vi "My Schedule vs Prins FIFO Scheduler with Plotting.vi"() -> ()   [LabVIEW 2013, in "Scheduler.lvclass"]
uses:
  Scheduler.lvclass
  Controls/GanntChart_Element.ctl
  Controls/GapStructure4FIFOEngine.ctl
  Controls/Prins FIFO Scheduler Result Cluster.ctl
  Operation to Machine Job Tuple.vi
  Check Other Machines for Schedule Time.vi
  Schedule Job.vi
  Find Gaps on Particular Machine.vi
  Increment Number of Jobs on Machine.vi
  Find Job On Other Machines.vi
  <vilib>/dlg_ctls.llb/Space Constant.vi
  <vilib>/Analysis/1siggen.llb/Riffle Array (I32).vi
  <vilib>/Heliosphere Research LLC/Advanced Plotting Toolkit/api_core/New.vi
  <vilib>/Heliosphere Research LLC/Advanced Plotting Toolkit/api_annotations/XLabel.vi
  <vilib>/Heliosphere Research LLC/Advanced Plotting Toolkit/api_figure/YTicks.vi
  <vilib>/Heliosphere Research LLC/Advanced Plotting Toolkit/api_figure/Grids.vi
  <vilib>/Heliosphere Research LLC/Advanced Plotting Toolkit/api_core/View.vi
  <vilib>/Heliosphere Research LLC/Advanced Plotting Toolkit/api_core/Close.vi
  <vilib>/Heliosphere Research LLC/Advanced Plotting Toolkit/api_figure/Limits.vi
  <vilib>/Heliosphere Research LLC/Advanced Plotting Toolkit/api_annotations/Rectangle.vi
  <vilib>/Heliosphere Research LLC/Advanced Plotting Toolkit/api_annotations/Text.vi
  <vilib>/Analysis/NI_AALBase.lvlib
panel:
  out "Total Tardiness (U16)":u16
  out "Nondelay Sch After":u16[](array[numeric])
  out "Nondelay After Reorder":picture
  out "Nondelay Before Reorder":picture
  out "error out":errorcluster
  in  "error in (no error)":errorcluster
  out "Schedule":u16[](array[numeric])
  out "Prins FIFO Scheduler":picture
  out "Start Times":i32[][](array[numeric])
  out "My Scheduler Result":picture
  out "Gannt Chart Out":T1[][](array[typedef])
  out "Completion Times":i32[][](array[numeric])
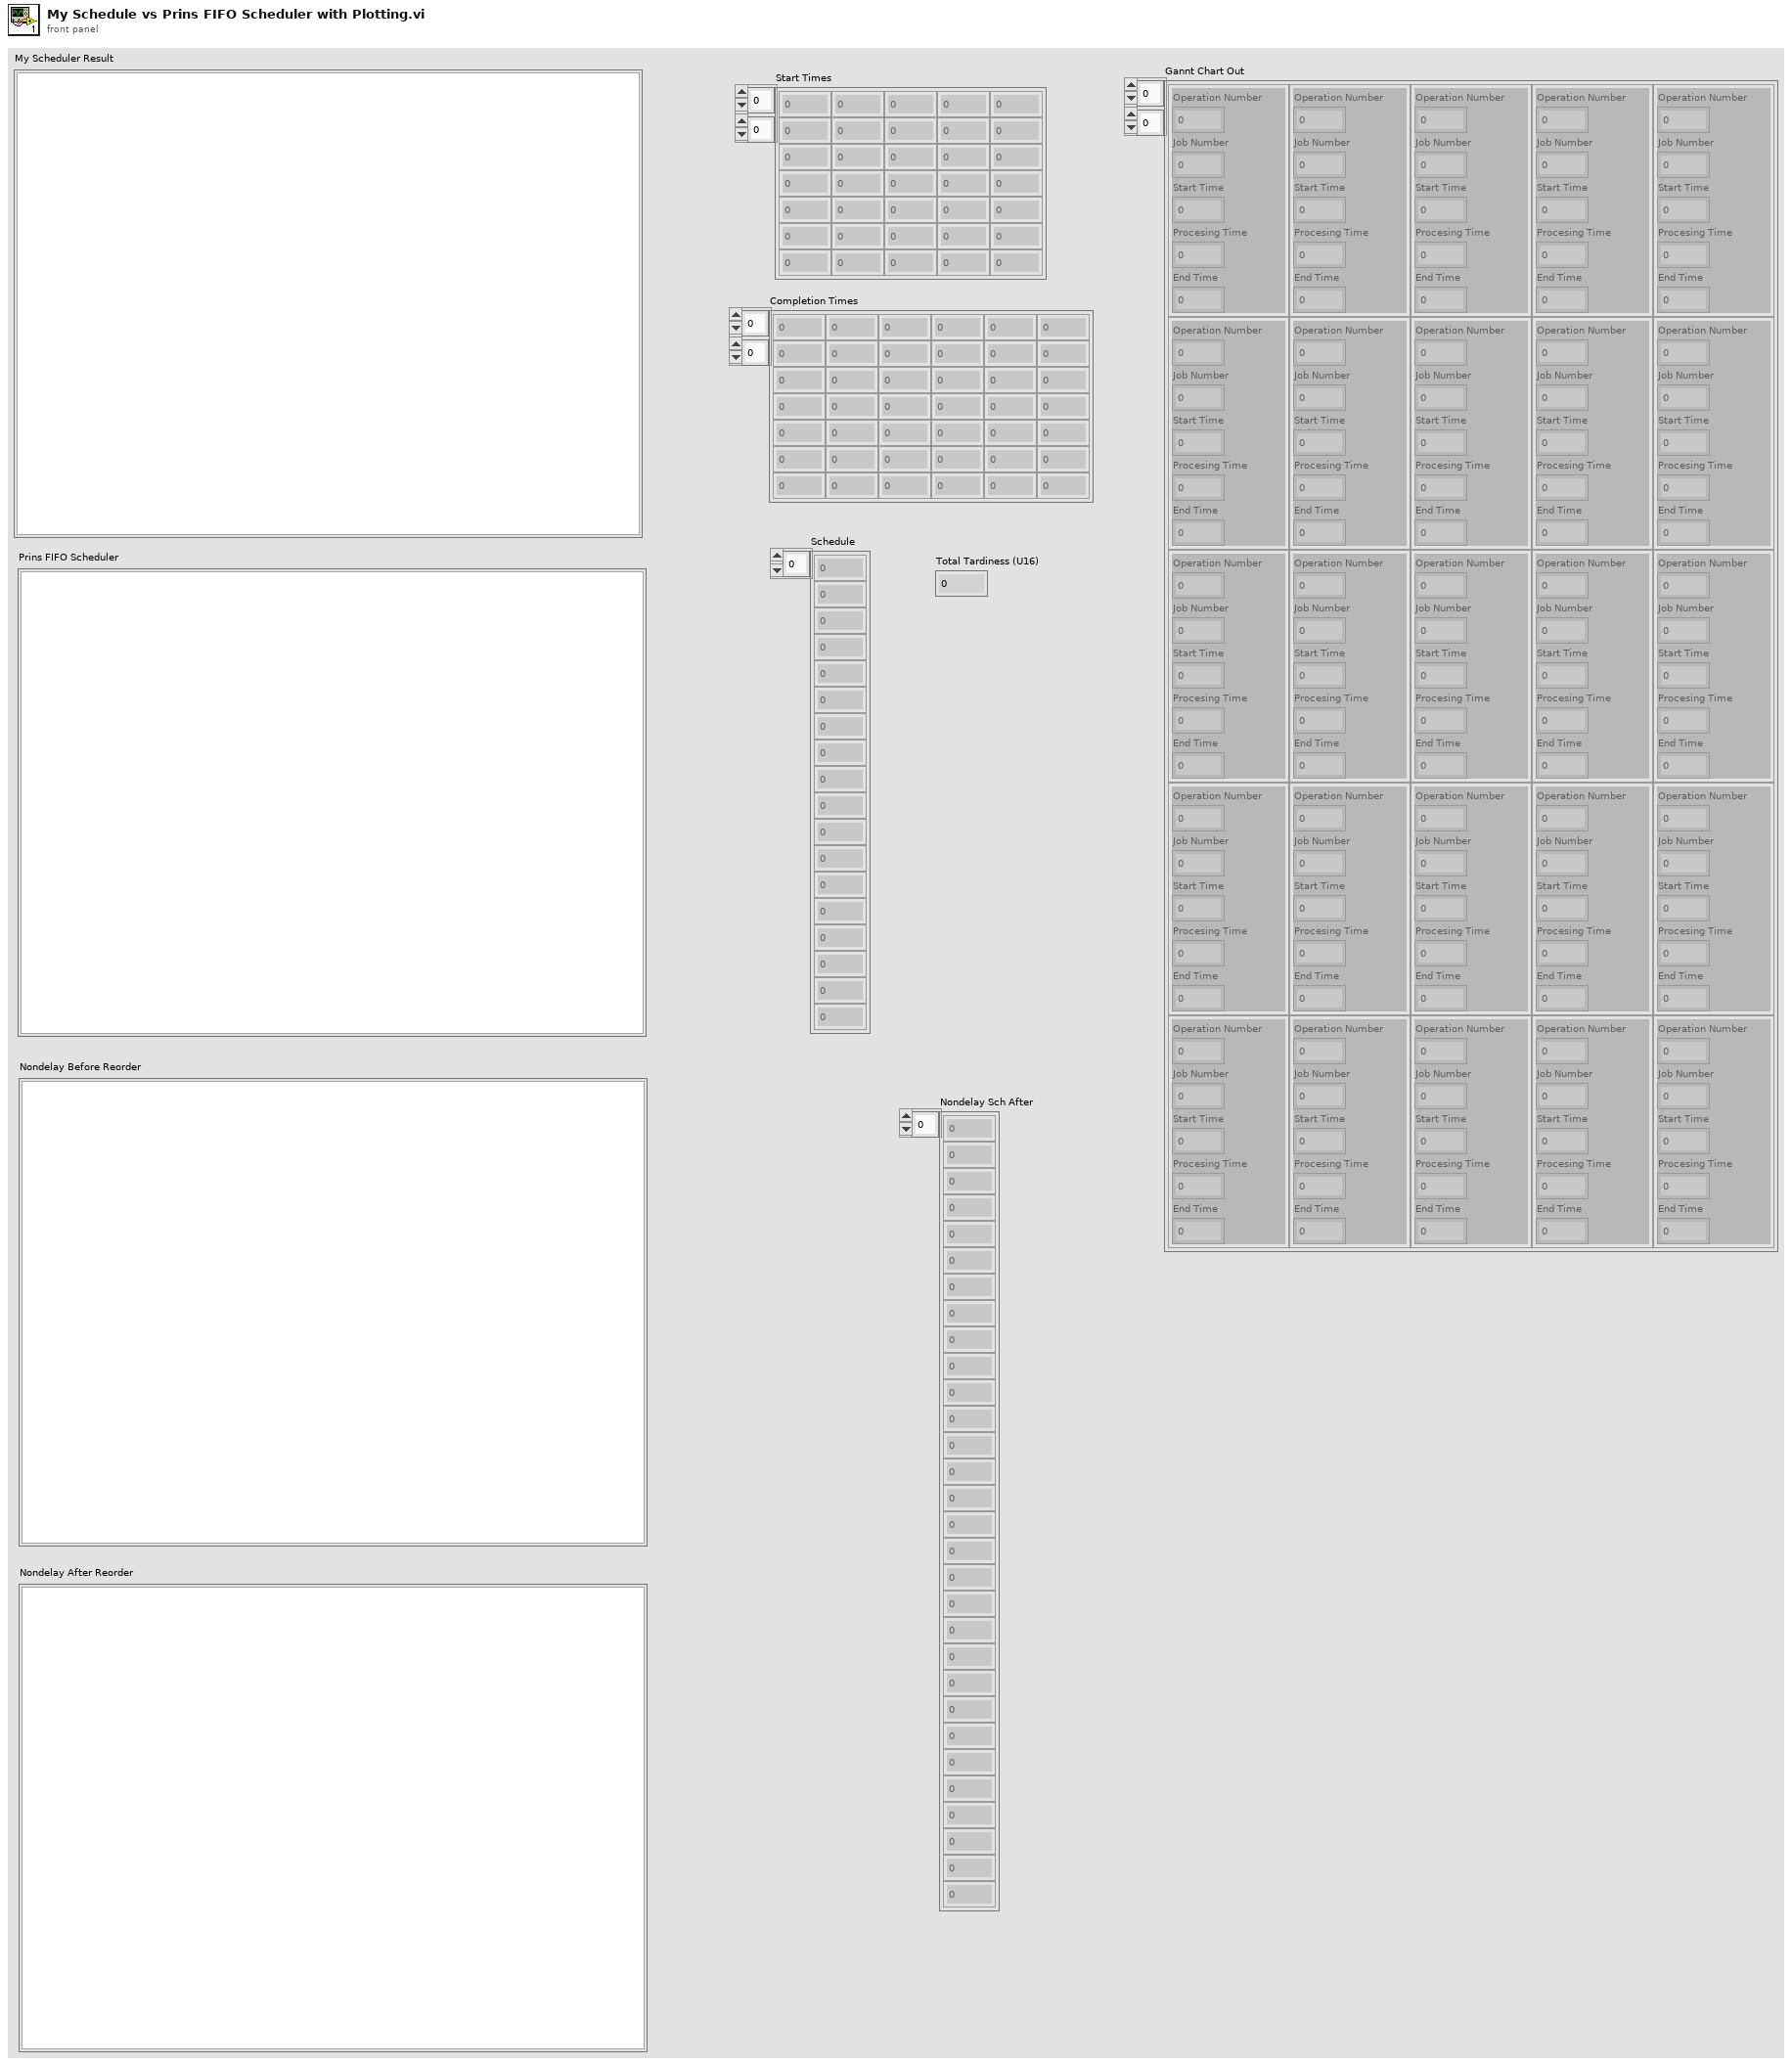
[diagram p1: front panel]
types:
  T1 = typedef "GanntChart_Element.ctl" = cluster{"Operation Number":i32, "Job Number":i32, "Start Time":i32, "Procesing Time":u16, "End Time":i32}
  T2 = typedef "Scheduler.lvclass/Prins FIFO Scheduler Result Cluster.ctl" = cluster{"Start Times":u16[][], "Completion Times":u16[][], "Processing Times":u16[][]}
  T3 = typedef "Scheduler.lvclass/GapStructure4FIFOEngine.ctl" = cluster{"Gap Start":i32, "Gap End":i32, "Gap Valid?":bool}
  T4 = typedef "Scheduler.lvclass/ValidGaps.ctl" = cluster{"Gap Start Time":i32, "Gap End Time":i32, "Gap Interval":i32}
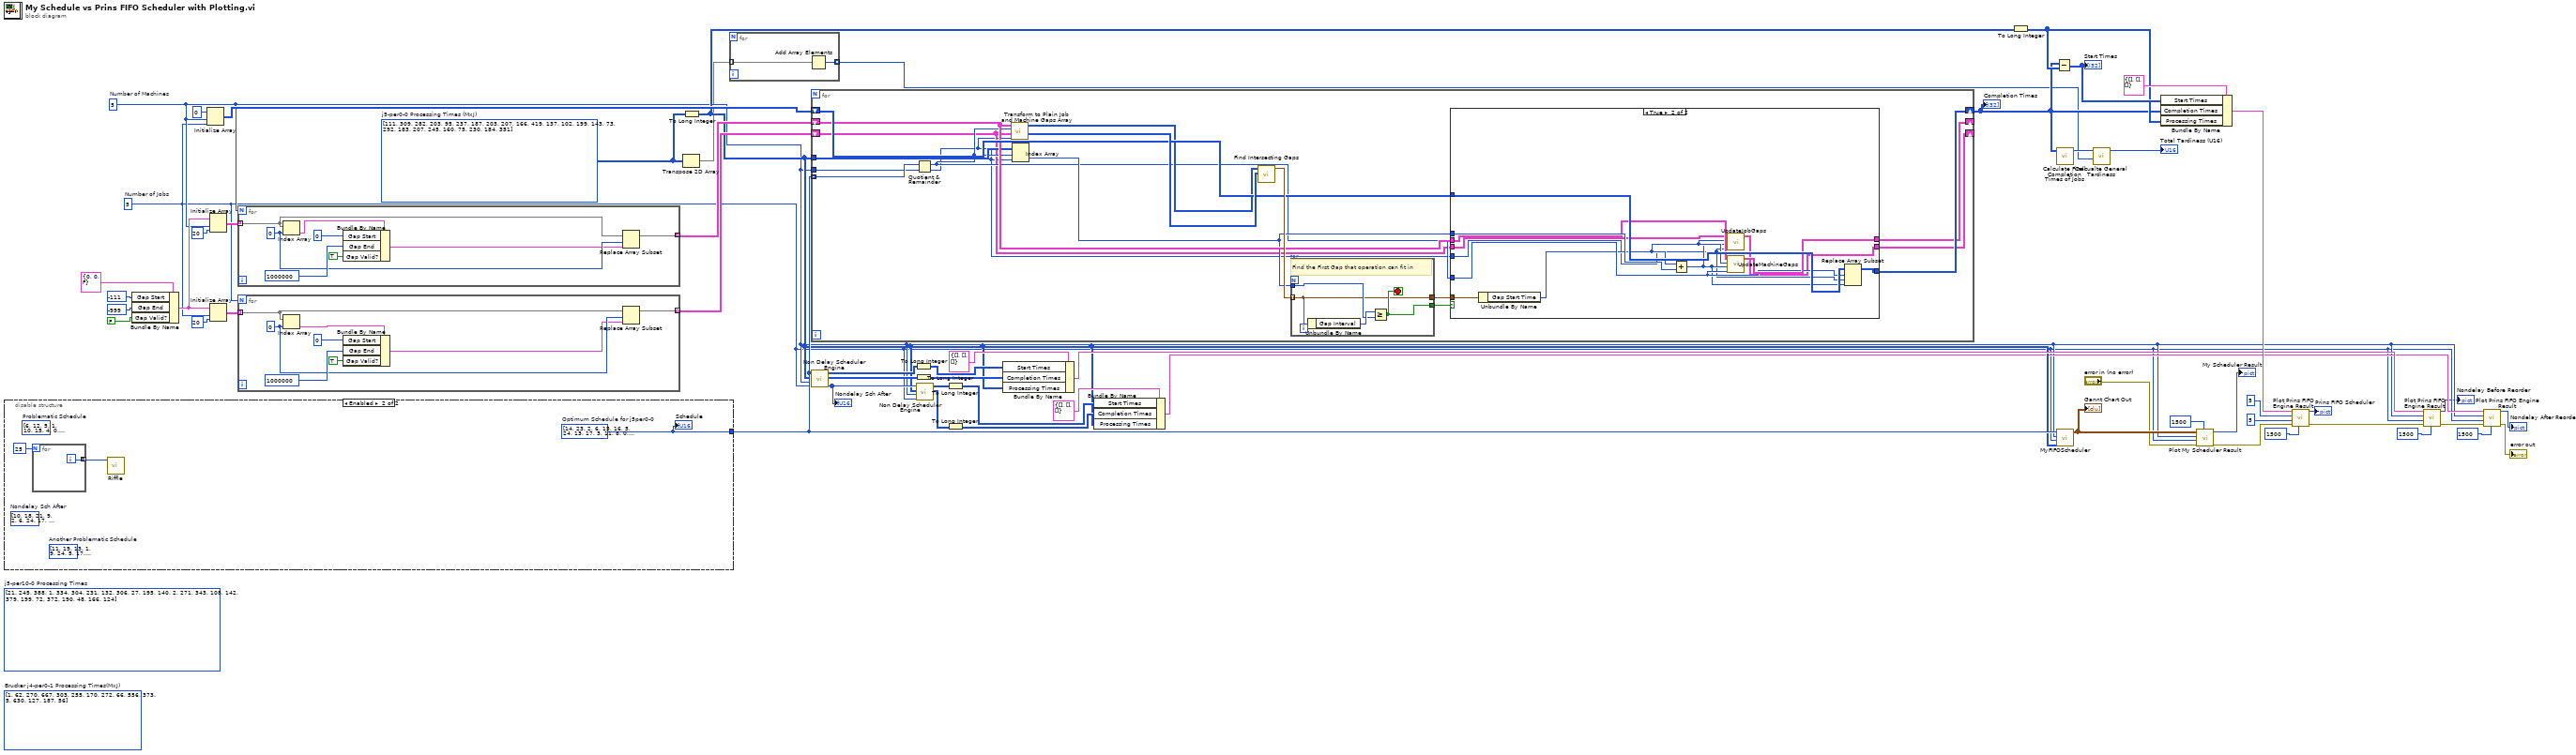
[diagram p0: block diagram]
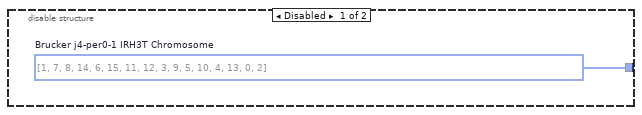
[diagram p2: hidden frame]
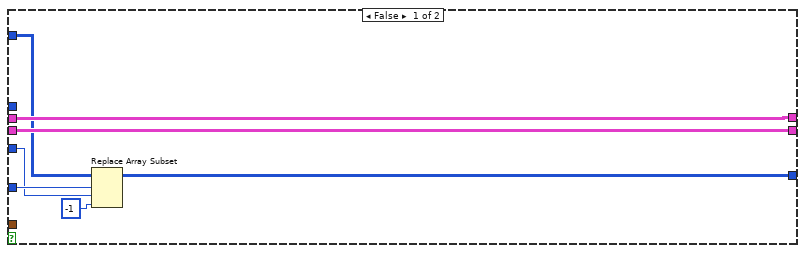
[diagram p3: hidden frame]
diagram:
  w4 = u16[][] [[111, 309, 282, 203, 95], [237, 187, 203, 207, 166], [419, 137, 102, 199, 143], [73, 292, 183, 207, 245], [160, 75, 230, 184, 351]]  # j5-per0-0 Processing Times (MxJ)
  (unwired) u16[][] [[21, 245, 388, 1, 334], [304, 231, 132, 306, 27], [195, 140, 2, 271, 343], [108, 142, 379, 199, 72], [372, 190, 48, 166, 124]]  # j5-per10-0 Processing Times
  (unwired) u16[][] [[1, 62, 270, 667], [303, 255, 170, 272], [66, 556, 373, 5], [630, 127, 187, 56]]  # Brucker j4-per0-1 Processing Times(MxJ)
  w14 = 5  # Number of Jobs
  w15 = 5  # Number of Machines
  n1 = disable-structure shown="Enabled" {
    disable-tunnel: [w57 w58] -> w30
    frame Disabled {
      w57 = i32[] [1, 7, 8, 14, 6, 15, 11, 12, 3, 9, 5, 10, 4, 13, 0, 2]  # Brucker j4-per0-1 IRH3T Chromosome
    }
    frame Enabled {
      w58 = u16[] [14, 23, 2, 6, 15, 16, 5, 24, 13, 17, 3, 11, 8, 0, 19, 20, 12, 1, 22, 10, 9, 18, 21, 4, 7]  # Optimum Schedule for j5per0-0
      (unwired) u16[] [10, 18, 21, 9, 2, 6, 24, 17, 3, 23, 4, 20, 13, 16, 7, 0, 22, 5, 14, 1, 19, 8, 15, 12, 11]  # Nondelay Sch After
      (unwired) u16[] [11, 19, 13, 1, 9, 24, 5, 17, 14, 0, 2, 8, 3, 6, 20, 4, 16, 18, 10, 23, 22, 15, 12, 7, 21]  # Another Problematic Schedule
      (unwired) i32[] [6, 12, 5, 1, 10, 15, 4, 0, 14, 7, 13, 3, 2, 8, 11, 9]  # Problematic Schedule
      n2 = for {
        N: 25 -> [_]
        tunnel: [w61] -> w60 mode=indexing
        i -> [w61]
      }
      n3 = call-poly <vilib>:"Riffle.vi"("X"=w60) -> ()  [unwired: 8 in, 3 out]
      "Schedule" <- w58
    }
  }
  n4 = Bundle By Name(cluster=T3 {"Gap Start"=0, "Gap End"=0, "Gap Valid?"=FALSE}, "Gap Start"=-111, "Gap End"=-999, "Gap Valid?"=FALSE) -> (w48:T3)
  n5 = Initialize Array(0, w15, w14) -> (w44:i32[][])
  n6 = Initialize Array(w48, w15, 20 ("dimension size")) -> (w47:T3[][])
  n7 = Initialize Array(w48, w14, 20 ("dimension size")) -> (w50:T3[][])
  n8 = for {
    N: w15 -> [_]
    tunnel: [w62] -> w46 mode=indexing
    tunnel: w47 -> [w65] mode=indexing
    w64 = 0 ("index")
    n9 = Index Array(array=w65, index=w64) -> (element=w69:T3)
    n10 = Bundle By Name(cluster=w69, "Gap Start"=0, "Gap End"=1000000, "Gap Valid?"=TRUE) -> (w63:T3)
    n11 = Replace Array Subset(array=w65, new element=w63, index=w64) -> (w62:T3[])
  }
  n12 = for {
    N: w14 -> [_]
    tunnel: [w70] -> w56 mode=indexing
    tunnel: w50 -> [w73] mode=indexing
    w72 = 0 ("index")
    n13 = Index Array(array=w73, index=w72) -> (element=w77:T3)
    n14 = Bundle By Name(cluster=w77, "Gap Start"=0, "Gap End"=1000000, "Gap Valid?"=TRUE) -> (w71:T3)
    n15 = Replace Array Subset(array=w73, new element=w71, index=w72) -> (w70:T3[])
  }
  n16 = Transpose 2D Array(2D array=w4) -> (transposed array=w3:u16[][])
  n17 = To Long Integer(number=w4) -> (32bit integer=w17:i32[][])
  n18 = for {
    tunnel: w3 -> [w79] mode=indexing
    tunnel: [w78] -> w2 mode=indexing
    n19 = Add Array Elements(numeric array=w79) -> (sum=w78:u16)
  }
  n20 = for {
    tunnel: w30 -> [w96] mode=indexing
    tunnel: w15 -> [w95]
    shift-right: [w89] -> w6
    shift-left: w44 -> [w90]
    tunnel: w17 -> [w85]
    shift-right: [w87] -> _
    shift-left: w46 -> [w88]
    shift-right: [w86] -> _
    shift-left: w56 -> [w81]
    n21 = Quotient & Remainder(x=w96, y=w95) -> (x-y*floor(x/y)=w82:i32, floor(x/y)=w80:i32)
    n22 = call "Transform to Plain Job and Machine Gaps Array.vi"("v"=w80, "Job Gaps"=w81, "u"=w82, "Machine Gaps"=w88) -> ("Job Gaps Array"=w94:i32[][], "Machine Gaps Array"=w83:i32[][])  [unwired: 6 in]
    n23 = Index Array(array=w85, index (row)=w82, index (col)=w80) -> (element=w84:i32)
    n24 = call "Find Intersecting Gaps.vi"("Job Gaps Array"=w94, "Machine Gaps Array"=w83) -> ("Gaps Array"=w93:T4[])  [unwired: 9 in]
    n25 = for {
      tunnel: w93 -> [w116] mode=indexing
      tunnel: w84 -> [w118]
      tunnel: [w117] -> w92
      tunnel: [w116] -> w91
      stop <- w117 stop-if-true
      # "Find the First Gap that operation can fit in"
      n26 = Unbundle By Name(w116) -> ("Gap Interval"=w119:i32)
      n27 = Greater Or Equal?(x=w119, y=w118) -> (x >= y?=w117:bool)
    }
    n28 = case shown="True" w92 {
      tunnel: w91 -> [_ w115]
      tunnel: w90 -> [w98 w114]
      tunnel: w82 -> [w101 w109]
      tunnel: w80 -> [w100 w106]
      tunnel: w84 -> [_ w113]
      tunnel: [w97 w112] -> w89
      tunnel: w88 -> [w103 w110]
      tunnel: [w103 w111] -> w87
      tunnel: w81 -> [w102 w105]
      tunnel: [w102 w104] -> w86
      frame False {
        n29 = Replace Array Subset(array=w98, new element=-1 ("new element/subarray"), index (row)=w101, index (col)=w100) -> (w97:i32[][])
      }
      frame True {
        n30 = Unbundle By Name(w115) -> ("Gap Start Time"=w108:i32)
        n31 = Add(x=w108, y=w113) -> (x+y=w107:i32)
        n32 = call "UpdateJobGaps.vi"("v( Job Index)"=w106, "Operation Finish Time"=w107, "Operation Start Time"=w108, "Job Gaps in"=w105) -> ("Job Gaps out"=w104:T3[][])  [unwired: 7 in]
        n33 = call "UpdateMachineGaps.vi"("u( Machine Index)"=w109, "Operation Finish Time"=w107, "Operation Start Time"=w108, "Machine Gaps in"=w110) -> ("Machine Gaps out"=w111:T3[][])  [unwired: 7 in]
        n34 = Replace Array Subset(array=w114, new element=w107, index (row)=w109, index (col)=w106) -> (w112:i32[][])
      }
    }
  }
  "Completion Times" <- w6
  n35 = call "Non Delay Scheduler Engine.vi"("Number of  Jobs"=w14, "Number of Machines"=w15, "Processing Times"=w17, "Schedule"=w30) -> ("Reordered Schedule"=w24:u16[], "Completion Times"=w26:u16[][], "Start Times"=w28:u16[][])  [unwired: 2 in, 3 out]
  "Nondelay Sch After" <- w24
  n36 = To Long Integer(number=w28) -> (32bit integer=w27:i32[][])
  n37 = To Long Integer(number=w26) -> (32bit integer=w25:i32[][])
  n38 = call "Non Delay Scheduler Engine.vi"("Number of  Jobs"=w14, "Number of Machines"=w15, "Processing Times"=w17, "Schedule"=w24) -> ("Completion Times"=w19:u16[][], "Start Times"=w21:u16[][])  [unwired: 2 in, 4 out]
  n39 = To Long Integer(number=w21) -> (32bit integer=w20:i32[][])
  n40 = To Long Integer(number=w19) -> (32bit integer=w18:i32[][])
  n41 = Bundle By Name(cluster=T2 {"Start Times"=[], "Completion Times"=[], "Processing Times"=[]}, "Start Times"=w27, "Completion Times"=w25, "Processing Times"=w17) -> (w23:T2)
  n42 = Bundle By Name(cluster=T2 {"Start Times"=[], "Completion Times"=[], "Processing Times"=[]}, "Start Times"=w20, "Completion Times"=w18, "Processing Times"=w17) -> (w16:T2)
  n43 = To Long Integer(number=w17) -> (32bit integer=w39:i32[][])
  n44 = Subtract(x=w6, y=w39) -> (x-y=w40:i32[][])
  "Start Times" <- w40
  n45 = call "Calculate Final Completion Times of Jobs.vi"("Completion Times (MxJ)"=w6) -> ("Job Completion Times"=w5:i32[])  [unwired: 10 in]
  n46 = call "MyFIFOScheduler.vi"("Processing Times (Rows Mach.Cols Jobs)"=w17, "Number of Jobs"=w14, "Number of Machines"=w15, "Schedule"=w30) -> ("Gannt Chart Out"=w42:T1[][])  [unwired: 6 in, 1 out]
  "Gannt Chart Out" <- w42
  n47 = call "Calcualte General Tardiness.vi"("Due Dates"=w2, "Job Completion Times"=w5) -> ("Total Tardiness (U16)"=→"Total Tardiness (U16)":u16)  [unwired: 9 in]
  n48 = Bundle By Name(cluster=T2 {"Start Times"=[], "Completion Times"=[], "Processing Times"=[]}, "Start Times"=w40, "Completion Times"=w6, "Processing Times"=w39) -> (w38:T2)
  n49 = call "Plot My Scheduler Result.vi"("Fitness Value"=1500 ("Number of Machines"), "error in (no error)"="error in (no error)", "Number of Jobs"=w14, "Number of Machines"=w15, "Gannt Chart In"=w42) -> ("error out"=w31:errorcluster, "My Scheduler Graph"=→"My Scheduler Result":picture)  [unwired: 5 in]
  n50 = call "Plot Prins FIFO Engine Result.vi"("Plot Max Value"=1500 ("Fitness Value"), "error in (no error)"=w31, "Number of Jobs"=5, "Number of Machines"=5, "FIFO Results"=w38) -> ("error out"=w9:errorcluster, "Graph Out"=→"Prins FIFO Scheduler":picture)  [unwired: 5 in]
  n51 = call "Plot Prins FIFO Engine Result.vi"("Plot Max Value"=1500, "error in (no error)"=w9, "Number of Jobs"=w14, "Number of Machines"=w15, "FIFO Results"=w23) -> ("error out"=w8:errorcluster, "Graph Out"=→"Nondelay Before Reorder":picture)  [unwired: 5 in]
  n52 = call "Plot Prins FIFO Engine Result.vi"("Plot Max Value"=1500, "error in (no error)"=w8, "Number of Jobs"=w14, "Number of Machines"=w15, "FIFO Results"=w16) -> ("error out"=→"error out":errorcluster, "Graph Out"=→"Nondelay After Reorder":picture)  [unwired: 5 in]
